vi "HEWH ANSI Display.vi"(5 "Calculation Type":string(combo), 7 "Stop Timer":dbl=1200.0 format="%#_13g", 8 "Error In":errorcluster, 9 "Software Elapsed Time":dbl, 11 "ANSI Rate In":T1) -> (0 "Error Out":errorcluster, 1 "Raw Timer":dbl, 2 "ANSI Display":string, 3 "ANSI Rate Out":T1)   [LabVIEW 2019]
uses:
  Range/Type Definitions/RANGE ANSI Rate.ctl
  Utility/Custom Pallet Controls/Custom Pallet Timer.ctl
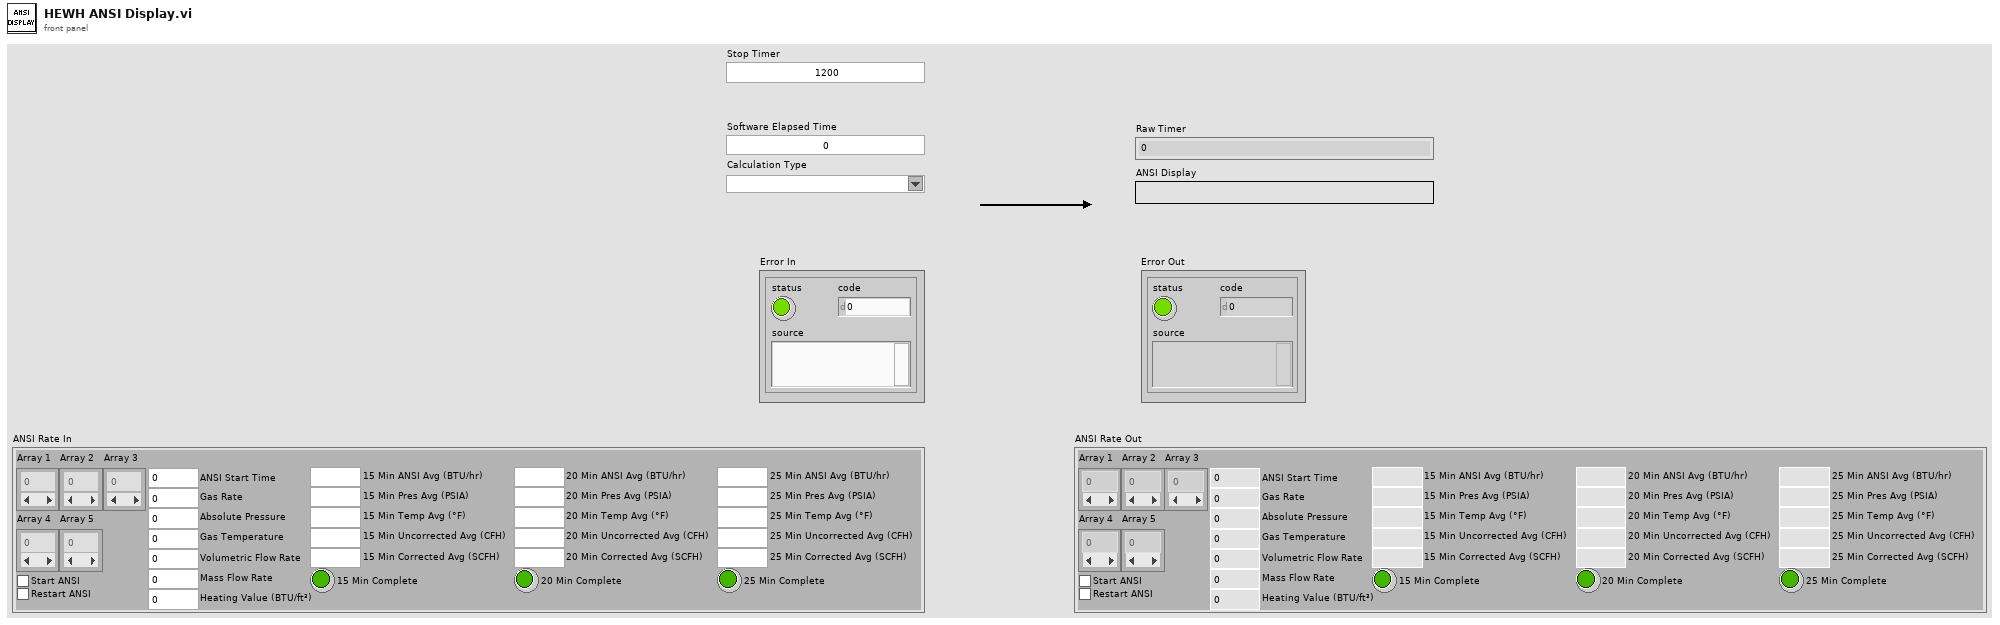
[diagram p1: front panel]
types:
  T1 = typedef "RANGE ANSI Rate.ctl" = cluster{"Array 1":dbl[], "Array 3":dbl[], "Array 2":dbl[], "Start ANSI":bool, "ANSI Start Time":dbl, "Restart ANSI":bool, "15 Min ANSI Avg (BTU/hr)":dbl, "20 Min ANSI Avg (BTU/hr)":dbl, "25 Min ANSI Avg (BTU/hr)":dbl, "Absolute Pressure":dbl, "Gas Temperature":dbl, "Volumetric Flow Rate":dbl, "Mass Flow Rate":dbl, "Array 4":dbl[], "Array 5":dbl[], "Gas Rate":dbl, "15 Min Pres Avg (PSIA)":dbl, "20 Min Pres Avg (PSIA)":dbl, "25 Min Pres Avg (PSIA)":dbl, "15 Min Temp Avg (°F) ":dbl, "20 Min Temp Avg (°F)":dbl, "25 Min Temp Avg (°F)":dbl, "15 Min Uncorrected Avg (CFH)":dbl, "20 Min Uncorrected Avg (CFH)":dbl, "25 Min Uncorrected Avg (CFH)":dbl, "15 Min Corrected Avg (SCFH)":dbl, "20 Min Corrected Avg (SCFH)":dbl, "25 Min Corrected Avg (SCFH)":dbl, "15 Min Complete":bool, "20 Min Complete":bool, "25 Min Complete":bool, "Heating Value (BTU/ft³)":dbl}
  T2 = typedef "Custom Pallet Timer.ctl" = dbl
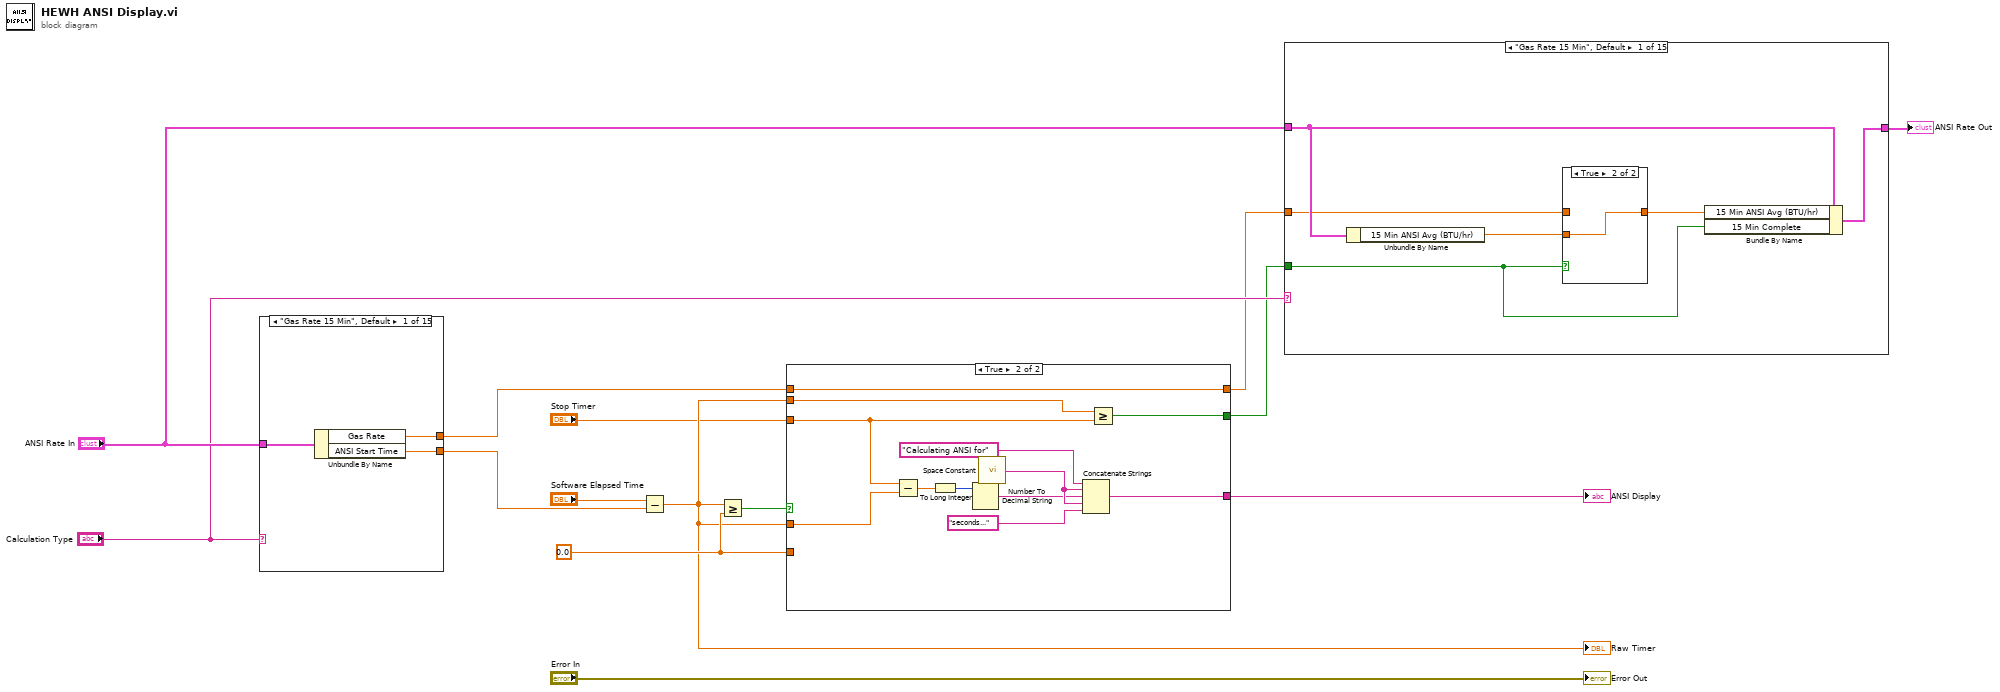
[diagram p0: block diagram]
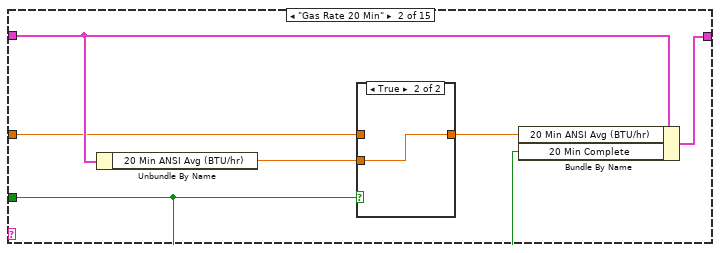
[diagram p3: hidden frame]
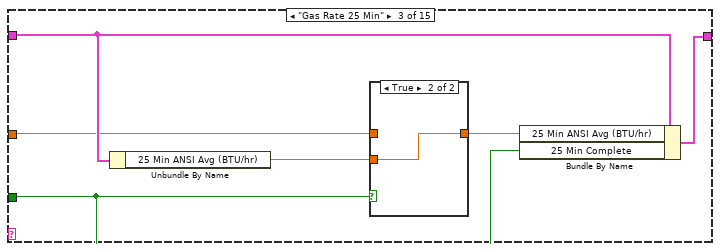
[diagram p5: hidden frame]
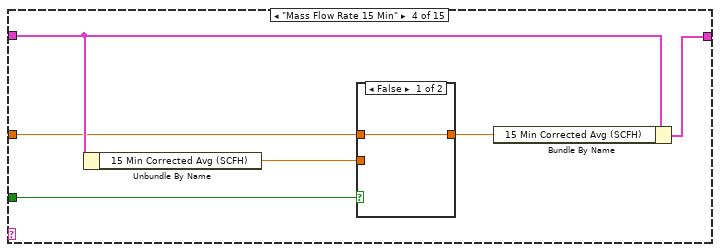
[diagram p7: hidden frame]
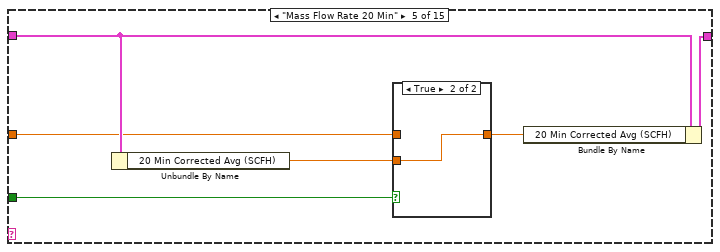
[diagram p9: hidden frame]
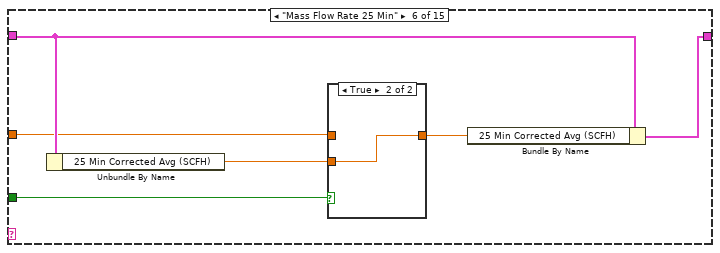
[diagram p11: hidden frame]
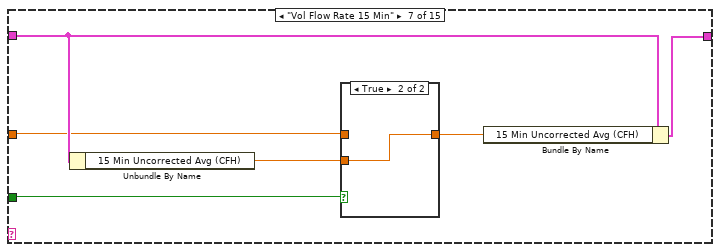
[diagram p13: hidden frame]
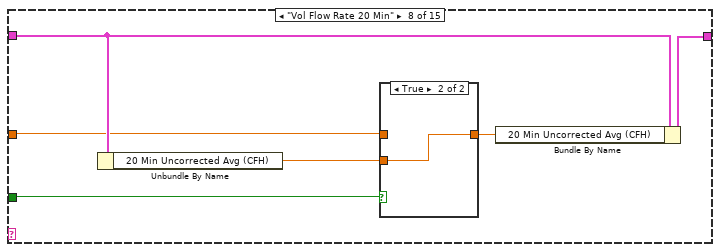
[diagram p15: hidden frame]
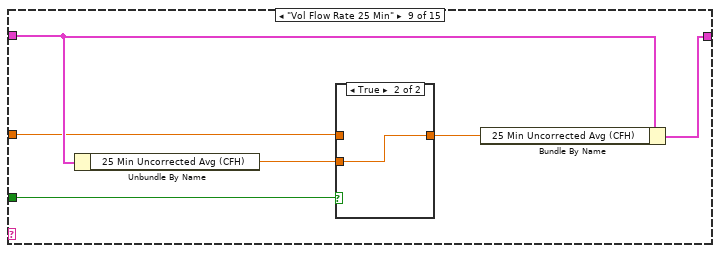
[diagram p17: hidden frame]
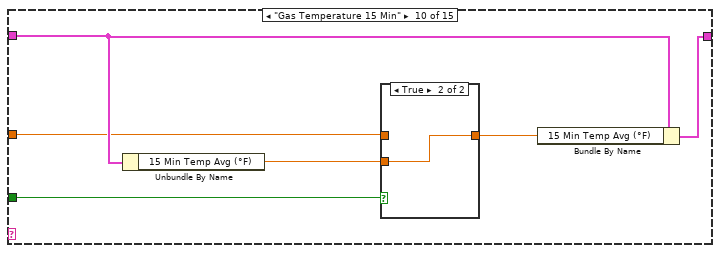
[diagram p19: hidden frame]
diagram:
  w10 = T2 0.0 ("y")
  n1 = case shown="\"Gas Rate 15 Min\", Default" "Calculation Type" {
    tunnel: "ANSI Rate In" -> [w17 w20 w23 w26 w29 w32 w35 w38 w41 w44 w47 w50 w53 w56 w59]
    tunnel: [w16 w18 w21 w24 w27 w30 w33 w36 w39 w42 w45 w48 w51 w54 w57] -> w7
    tunnel: [w15 w19 w22 w25 w28 w31 w34 w37 w40 w43 w46 w49 w52 w55 w58] -> w6
    frame "Gas Rate 15 Min", Default {
      n2 = Unbundle By Name(w17) -> ("Gas Rate"=w15:dbl, "ANSI Start Time"=w16:dbl)
    }
    frame "Gas Rate 20 Min" {
      n3 = Unbundle By Name(w20) -> ("Gas Rate"=w19:dbl, "ANSI Start Time"=w18:dbl)
    }
    frame "Gas Rate 25 Min" {
      n4 = Unbundle By Name(w23) -> ("Gas Rate"=w22:dbl, "ANSI Start Time"=w21:dbl)
    }
    frame "Mass Flow Rate 15 Min" {
      n5 = Unbundle By Name(w26) -> ("Mass Flow Rate"=w25:dbl, "ANSI Start Time"=w24:dbl)
    }
    frame "Mass Flow Rate 20 Min" {
      n6 = Unbundle By Name(w29) -> ("Mass Flow Rate"=w28:dbl, "ANSI Start Time"=w27:dbl)
    }
    frame "Mass Flow Rate 25 Min" {
      n7 = Unbundle By Name(w32) -> ("Mass Flow Rate"=w31:dbl, "ANSI Start Time"=w30:dbl)
    }
    frame "Vol Flow Rate 15 Min" {
      n8 = Unbundle By Name(w35) -> ("Volumetric Flow Rate"=w34:dbl, "ANSI Start Time"=w33:dbl)
    }
    frame "Vol Flow Rate 20 Min" {
      n9 = Unbundle By Name(w38) -> ("Volumetric Flow Rate"=w37:dbl, "ANSI Start Time"=w36:dbl)
    }
    frame "Vol Flow Rate 25 Min" {
      n10 = Unbundle By Name(w41) -> ("Volumetric Flow Rate"=w40:dbl, "ANSI Start Time"=w39:dbl)
    }
    frame "Gas Temperature 15 Min" {
      n11 = Unbundle By Name(w44) -> ("Gas Temperature"=w43:dbl, "ANSI Start Time"=w42:dbl)
    }
    frame "Gas Temperature 20 Min" {
      n12 = Unbundle By Name(w47) -> ("Gas Temperature"=w46:dbl, "ANSI Start Time"=w45:dbl)
    }
    frame "Gas Temperature 25 Min" {
      n13 = Unbundle By Name(w50) -> ("Gas Temperature"=w49:dbl, "ANSI Start Time"=w48:dbl)
    }
    frame "Gas Pressure 15 Min" {
      n14 = Unbundle By Name(w53) -> ("Absolute Pressure"=w52:dbl, "ANSI Start Time"=w51:dbl)
    }
    frame "Gas Pressure 20 Min" {
      n15 = Unbundle By Name(w56) -> ("Absolute Pressure"=w55:dbl, "ANSI Start Time"=w54:dbl)
    }
    frame "Gas Pressure 25 Min" {
      n16 = Unbundle By Name(w59) -> ("Absolute Pressure"=w58:dbl, "ANSI Start Time"=w57:dbl)
    }
  }
  n17 = Subtract(x="Software Elapsed Time", y=w7) -> (x-y=w9:dbl)
  "Raw Timer" <- w9
  n18 = Greater Or Equal?(x=w9, y=w10) -> (x >= y?=w12:bool)
  n19 = case shown="True" w12 {
    tunnel: w6 -> [_ w82]
    tunnel: [0.0 ("ANSI Average (BTU/hr) Input") w82] -> w2
    tunnel: [w65 w75] -> w11
    tunnel: w10 -> [w63 _]
    tunnel: w9 -> [w62 w74]
    tunnel: w9 -> [_ w73]
    tunnel: [FALSE w72] -> w1
    tunnel: "Stop Timer" -> [_ w71]
    frame False {
      n20 = Subtract(x=w63, y=w62) -> (x-y=w61:T2)
      n21 = To Long Integer(number=w61) -> (32bit integer=w64:i32)
      n22 = Number To Decimal String(number=w64) -> (decimal integer string=w67:string)  [unwired: 1 in]
      n23 = call <vilib>:"Space Constant.vi"() -> ("String"=w68:string)
      n24 = Concatenate Strings("Stabilizing ANSI for", w68, w67, w68, "seconds..." ("string")) -> (w65:string)
    }
    frame True {
      n25 = Subtract(x=w71, y=w74) -> (x-y=w76:dbl)
      n26 = To Long Integer(number=w76) -> (32bit integer=w77:i32)
      n27 = Number To Decimal String(number=w77) -> (decimal integer string=w79:string)  [unwired: 1 in]
      n28 = call <vilib>:"Space Constant.vi"() -> ("String"=w80:string)
      n29 = Concatenate Strings("Calculating ANSI for", w80, w79, w80, "seconds..." ("string")) -> (w75:string)
      n30 = Greater Or Equal?(x=w73, y=w71) -> (x >= y?=w72:bool)
    }
  }
  "ANSI Display" <- w11
  n31 = case shown="\"Gas Rate 15 Min\", Default" "Calculation Type" {
    tunnel: [w86 w93 w100 w110 w118 w126 w134 w142 w149 w157 w165 w173 w181 w189 w197] -> w5
    tunnel: "ANSI Rate In" -> [w85 w94 w102 w109 w117 w125 w133 w141 w150 w158 w166 w174 w182 w190 w198]
    tunnel: w2 -> [w84 w92 w101 w108 w116 w124 w132 w140 w148 w156 w164 w172 w180 w188 w196]
    tunnel: w1 -> [w83 w91 w99 w107 w115 w123 w131 w139 w147 w155 w163 w171 w179 w187 w195]
    frame "Gas Rate 15 Min", Default {
      n32 = Unbundle By Name(w85) -> ("15 Min ANSI Avg (BTU/hr)"=w88:dbl)
      n33 = case shown="True" w83 {
        tunnel: w88 -> [_ w90]
        tunnel: [w89 w90] -> w87
        tunnel: w84 -> [w89 _]
        frame False {
        }
        frame True {
        }
      }
      n34 = Bundle By Name(cluster=w85, "15 Min ANSI Avg (BTU/hr)"=w87, "15 Min Complete"=w83) -> (w86:T1)
    }
    frame "Gas Rate 20 Min" {
      n35 = Unbundle By Name(w94) -> ("20 Min ANSI Avg (BTU/hr)"=w96:dbl)
      n36 = case shown="True" w91 {
        tunnel: w96 -> [_ w98]
        tunnel: [w97 w98] -> w95
        tunnel: w92 -> [w97 _]
        frame False {
        }
        frame True {
        }
      }
      n37 = Bundle By Name(cluster=w94, "20 Min ANSI Avg (BTU/hr)"=w95, "20 Min Complete"=w91) -> (w93:T1)
    }
    frame "Gas Rate 25 Min" {
      n38 = Unbundle By Name(w102) -> ("25 Min ANSI Avg (BTU/hr)"=w104:dbl)
      n39 = case shown="True" w99 {
        tunnel: w104 -> [_ w106]
        tunnel: [w105 w106] -> w103
        tunnel: w101 -> [w105 _]
        frame False {
        }
        frame True {
        }
      }
      n40 = Bundle By Name(cluster=w102, "25 Min ANSI Avg (BTU/hr)"=w103, "25 Min Complete"=w99) -> (w100:T1)
    }
    frame "Mass Flow Rate 15 Min" {
      n41 = Unbundle By Name(w109) -> ("15 Min Corrected Avg (SCFH)"=w112:dbl)
      n42 = case shown="False" w107 {
        tunnel: w112 -> [_ w114]
        tunnel: [w113 w114] -> w111
        tunnel: w108 -> [w113 _]
        frame False {
        }
        frame True {
        }
      }
      n43 = Bundle By Name(cluster=w109, "15 Min Corrected Avg (SCFH)"=w111) -> (w110:T1)
    }
    frame "Mass Flow Rate 20 Min" {
      n44 = Unbundle By Name(w117) -> ("20 Min Corrected Avg (SCFH)"=w120:dbl)
      n45 = case shown="True" w115 {
        tunnel: w120 -> [_ w122]
        tunnel: [w121 w122] -> w119
        tunnel: w116 -> [w121 _]
        frame False {
        }
        frame True {
        }
      }
      n46 = Bundle By Name(cluster=w117, "20 Min Corrected Avg (SCFH)"=w119) -> (w118:T1)
    }
    frame "Mass Flow Rate 25 Min" {
      n47 = Unbundle By Name(w125) -> ("25 Min Corrected Avg (SCFH)"=w128:dbl)
      n48 = case shown="True" w123 {
        tunnel: w128 -> [_ w130]
        tunnel: [w129 w130] -> w127
        tunnel: w124 -> [w129 _]
        frame False {
        }
        frame True {
        }
      }
      n49 = Bundle By Name(cluster=w125, "25 Min Corrected Avg (SCFH)"=w127) -> (w126:T1)
    }
    frame "Vol Flow Rate 15 Min" {
      n50 = Unbundle By Name(w133) -> ("15 Min Uncorrected Avg (CFH)"=w136:dbl)
      n51 = case shown="True" w131 {
        tunnel: w136 -> [_ w138]
        tunnel: [w137 w138] -> w135
        tunnel: w132 -> [w137 _]
        frame False {
        }
        frame True {
        }
      }
      n52 = Bundle By Name(cluster=w133, "15 Min Uncorrected Avg (CFH)"=w135) -> (w134:T1)
    }
    frame "Vol Flow Rate 20 Min" {
      n53 = Unbundle By Name(w141) -> ("20 Min Uncorrected Avg (CFH)"=w144:dbl)
      n54 = case shown="True" w139 {
        tunnel: w144 -> [_ w146]
        tunnel: [w145 w146] -> w143
        tunnel: w140 -> [w145 _]
        frame False {
        }
        frame True {
        }
      }
      n55 = Bundle By Name(cluster=w141, "20 Min Uncorrected Avg (CFH)"=w143) -> (w142:T1)
    }
    frame "Vol Flow Rate 25 Min" {
      n56 = Unbundle By Name(w150) -> ("25 Min Uncorrected Avg (CFH)"=w152:dbl)
      n57 = case shown="True" w147 {
        tunnel: w152 -> [_ w154]
        tunnel: [w153 w154] -> w151
        tunnel: w148 -> [w153 _]
        frame False {
        }
        frame True {
        }
      }
      n58 = Bundle By Name(cluster=w150, "25 Min Uncorrected Avg (CFH)"=w151) -> (w149:T1)
    }
    frame "Gas Temperature 15 Min" {
      n59 = Unbundle By Name(w158) -> ("15 Min Temp Avg (°F)"=w160:dbl)
      n60 = case shown="True" w155 {
        tunnel: w160 -> [_ w162]
        tunnel: [w161 w162] -> w159
        tunnel: w156 -> [w161 _]
        frame False {
        }
        frame True {
        }
      }
      n61 = Bundle By Name(cluster=w158, "15 Min Temp Avg (°F)"=w159) -> (w157:T1)
    }
    frame "Gas Temperature 20 Min" {
      n62 = Unbundle By Name(w166) -> ("20 Min Temp Avg (°F)"=w168:dbl)
      n63 = case shown="True" w163 {
        tunnel: w168 -> [_ w170]
        tunnel: [w169 w170] -> w167
        tunnel: w164 -> [w169 _]
        frame False {
        }
        frame True {
        }
      }
      n64 = Bundle By Name(cluster=w166, "20 Min Temp Avg (°F)"=w167) -> (w165:T1)
    }
    frame "Gas Temperature 25 Min" {
      n65 = Unbundle By Name(w174) -> ("25 Min Temp Avg (°F)"=w176:dbl)
      n66 = case shown="True" w171 {
        tunnel: w176 -> [_ w178]
        tunnel: [w177 w178] -> w175
        tunnel: w172 -> [w177 _]
        frame False {
        }
        frame True {
        }
      }
      n67 = Bundle By Name(cluster=w174, "25 Min Temp Avg (°F)"=w175) -> (w173:T1)
    }
    frame "Gas Pressure 15 Min" {
      n68 = Unbundle By Name(w182) -> ("15 Min Pres Avg (PSIA)"=w184:dbl)
      n69 = case shown="True" w179 {
        tunnel: w184 -> [_ w186]
        tunnel: [w185 w186] -> w183
        tunnel: w180 -> [w185 _]
        frame False {
        }
        frame True {
        }
      }
      n70 = Bundle By Name(cluster=w182, "15 Min Pres Avg (PSIA)"=w183) -> (w181:T1)
    }
    frame "Gas Pressure 20 Min" {
      n71 = Unbundle By Name(w190) -> ("20 Min Pres Avg (PSIA)"=w192:dbl)
      n72 = case shown="True" w187 {
        tunnel: w192 -> [_ w194]
        tunnel: [w193 w194] -> w191
        tunnel: w188 -> [w193 _]
        frame False {
        }
        frame True {
        }
      }
      n73 = Bundle By Name(cluster=w190, "20 Min Pres Avg (PSIA)"=w191) -> (w189:T1)
    }
    frame "Gas Pressure 25 Min" {
      n74 = Unbundle By Name(w198) -> ("25 Min Pres Avg (PSIA)"=w200:dbl)
      n75 = case shown="True" w195 {
        tunnel: w200 -> [_ w202]
        tunnel: [w201 w202] -> w199
        tunnel: w196 -> [w201 _]
        frame False {
        }
        frame True {
        }
      }
      n76 = Bundle By Name(cluster=w198, "25 Min Pres Avg (PSIA)"=w199) -> (w197:T1)
    }
  }
  "ANSI Rate Out" <- w5
  "Error Out" <- "Error In"
